vi "Calculate Buffer for Decimation.vi"(0 "Waveform Size In (100)":i32=100, 5 "Actual Points (1000)":i32=1000, 9 "Bytes of Each Point (1)":u8=1, 11 "error in (no error)":errorcluster) -> (4 "Waveform Size Out":i32, 6 "Number of Bytes per Chunck":i32, 8 "Number of Bytes per Fetch":i32, 10 "Decimation Buffer Size":i32, 15 "error out":errorcluster)   [LabVIEW 2013, in "Agilent 90000 Series.lvlib"]
doc: "Calculates total waveform points, chunk bytes, read buffer size, decimation buffer size by specified waveform size, actual points and bytes of each point."
uses:
  Agilent 90000 Series.lvlib
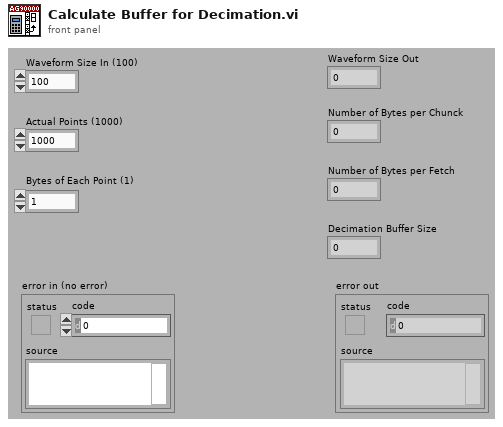
[diagram p1: front panel]
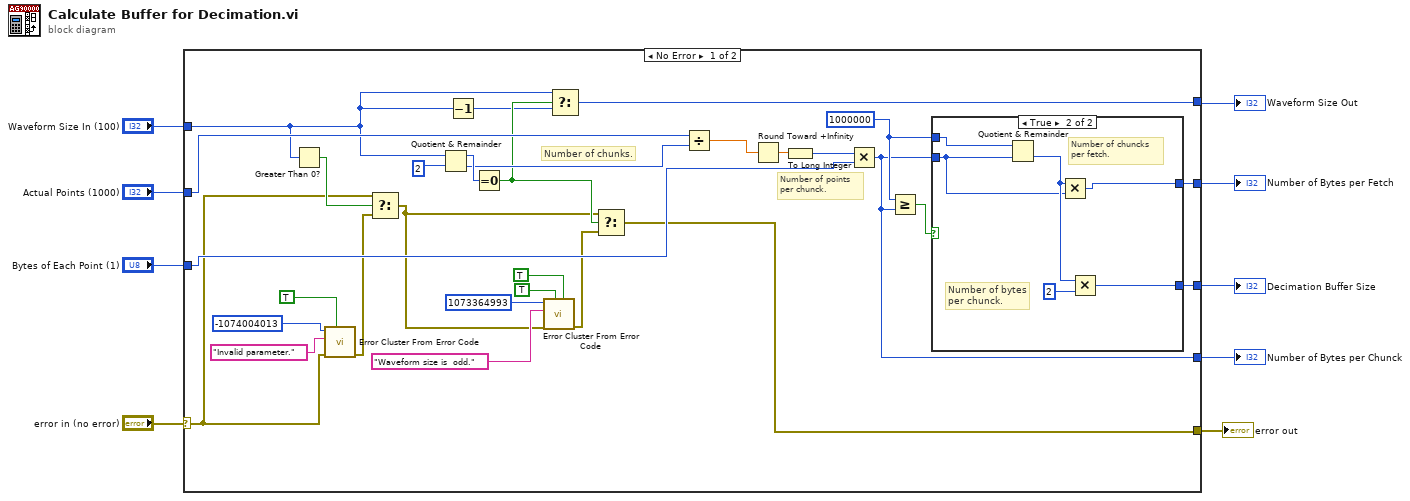
[diagram p0: block diagram]
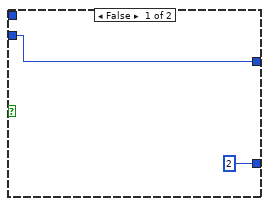
[diagram p2: hidden frame]
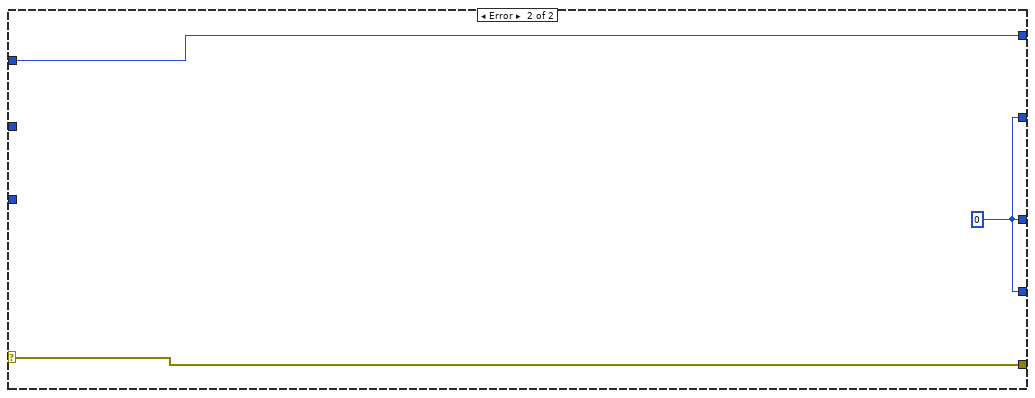
[diagram p3: hidden frame]
diagram:
  n1 = case shown="No Error" "error in (no error)" {
    selector: "error in (no error)" -> [w10 w50]
    tunnel: "Actual Points (1000)" -> [w39 _]
    tunnel: [w20 w49] -> w8
    tunnel: [w38 w49] -> w7
    tunnel: [w37 w49] -> w6
    tunnel: "Waveform Size In (100)" -> [w15 w48]
    tunnel: "Bytes of Each Point (1)" -> [w36 _]
    tunnel: [w28 w50] -> w2
    tunnel: [w22 w48] -> w1
    frame No Error {
      w21 = 1000000 ("x")
      # "Number of points\nper chunck."
      # "Number of chunks."
      n2 = Greater Than 0?(x=w15) -> (x > 0?=w14:bool)
      n3 = call <vilib>:"Error Cluster From Error Code.vi"("show call chain? (False)"=TRUE, "error in (no error)"=w10, "error message (\"\")"="Invalid parameter." ("error message (\"\")"), "error code (0)"=-1074004013) -> ("error out"=w13:errorcluster)  [unwired: 5 in]
      n4 = Select(t=w10, s=w14, f=w13) -> (s? t:f=w11:errorcluster)
      n5 = Quotient & Remainder(x=w15, y=2) -> (x-y*floor(x/y)=w34:i32, floor(x/y)=w29:i32)
      n6 = Decrement(x=w15) -> (x-1=w23:i32)
      n7 = Equal To 0?(x=w34) -> (x = 0?=w24:bool)
      n8 = call <vilib>:"Error Cluster From Error Code.vi"("is warning? (False)"=TRUE, "show call chain? (False)"=TRUE, "error in (no error)"=w11, "error message (\"\")"="Waveform size is  odd." ("error message (\"\")"), "error code (0)"=1073364993) -> ("error out"=w30:errorcluster)  [unwired: 4 in]
      n9 = Select(t=w15, s=w24, f=w23) -> (s? t:f=w22:i32)
      n10 = Select(t=w11, s=w24, f=w30) -> (s? t:f=w28:errorcluster)
      n11 = Divide(x=w39, y=w29) -> (x/y=w25:dbl)
      n12 = Round Toward +Infinity ("Round To +Infinity")(x=w25) -> (ceil(x): smallest int >= x=w26:dbl)
      n13 = To Long Integer(number=w26) -> (32bit integer=w27:i32)
      n14 = Multiply(x=w27, y=w36) -> (x*y=w20:i32)
      n15 = Greater Or Equal?(x=w21, y=w20) -> (x >= y?=w19:bool)
      n16 = case shown="True" w19 {
        tunnel: [2 w47] -> w38
        tunnel: [w41 w46] -> w37
        tunnel: w21 -> [_ w43]
        tunnel: w20 -> [w41 w42]
        frame False {
        }
        frame True {
          # "Number of chuncks\nper fetch."
          # "Number of bytes\nper chunck."
          n17 = Quotient & Remainder(x=w43, y=w42) -> (floor(x/y)=w44:i32)  [unwired: 1 out]
          n18 = Multiply(x=w44, y=w42) -> (x*y=w46:i32)
          n19 = Multiply(x=w44, y=2) -> (x*y=w47:i32)
        }
      }
    }
    frame Error {
      w49 = 0
    }
  }
  "Number of Bytes per Chunck" <- w8
  "Decimation Buffer Size" <- w7
  "Number of Bytes per Fetch" <- w6
  "error out" <- w2
  "Waveform Size Out" <- w1
